vi "array.vi"() -> ()   [LabVIEW 2018]
uses:
  global.vi
panel:
  out "appended array":i32[](array[numeric])
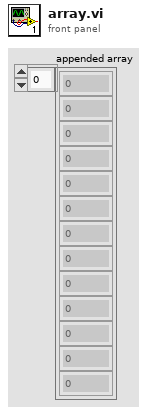
[diagram p1: front panel]
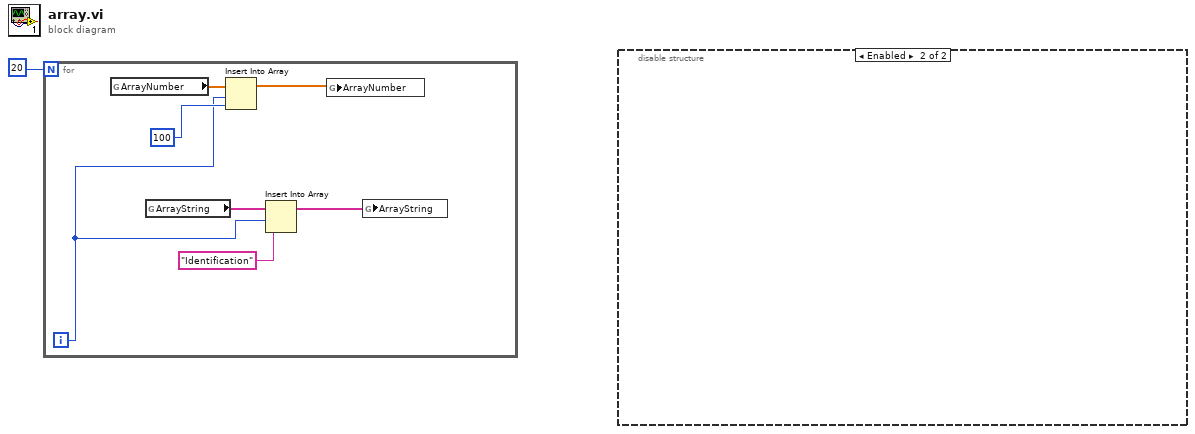
[diagram p0: block diagram]
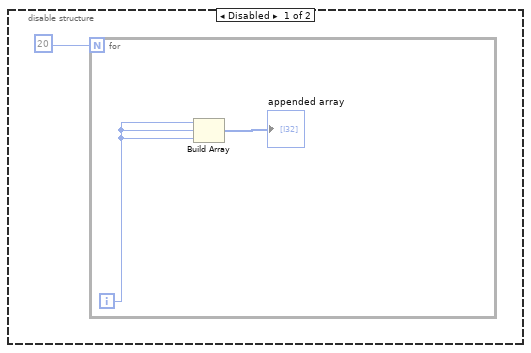
[diagram p2: hidden frame]
diagram:
  n1 = for {
    N: 20 -> [_]
    i -> [w2]
    n2 = global read "global.vi" "ArrayNumber"() -> (w8:dbl[])
    n3 = global read "global.vi" "ArrayString"() -> (w5:string[])
    n4 = Insert Into Array(array=w8, index=w2, new element=100) -> (w7:dbl[])
    n5 = Insert Into Array(array=w5, index=w2, new element="Identification") -> (w4:string[])
    n6 = global write "global.vi" "ArrayNumber"(w7) -> ()
    n7 = global write "global.vi" "ArrayString"(w4) -> ()
  }
  n8 = disable-structure shown="Enabled" {
    frame Disabled {
      n9 = for {
        N: 20 -> [_]
        i -> [w11]
        n10 = Build Array(w11, w11, w11) -> (→"appended array":i32[])
      }
    }
    frame Enabled {
    }
  }
